vi "Disconnect PV.vi"(8 "Error In":errorcluster, 10 "PV URL":string, 11 "BNT_SLTagMonitor in":refnum<class "BNT_SLTagMonitor.lvclass">) -> (0 "Error Out":errorcluster, 3 "BNT_SLTagMonitor out":refnum<class "BNT_SLTagMonitor.lvclass">)   [LabVIEW 2019, in "BNT_SLTagMonitor.lvlib" / "BNT_SLTagMonitor.lvclass"]
doc: "Close connection to process variable."
uses:
  BNT_SLTagMonitor.lvclass
  CSPP_Core/Actors/CSPP_PVMonitor/CSPP_PVMonitor.lvclass
  <vilib>/Skyline/Tag/Wrapper/Wrapper_class/NI Skyline Tag.lvclass
  <vilib>/Skyline/Tag/Wrapper/Wrapper_class/Close Tag (Single).vi
  C:/Users/Holger/Documents/LVP/CSPP/CSPP-Template/Packages/CSPP_Core/Actors/CSPP_PVMonitor/CSPP_PVMonitor.lvclass
  C:/Users/Holger/Documents/LVP/CSPP/CSPP-Template/Packages/CSPP_Core/Actors/CSPP_BaseActor/CSPP_BaseActor.lvclass
  C:/Program Files (x86)/National Instruments/LabVIEW 2019/vi.lib/ActorFramework/Actor/Actor.lvclass
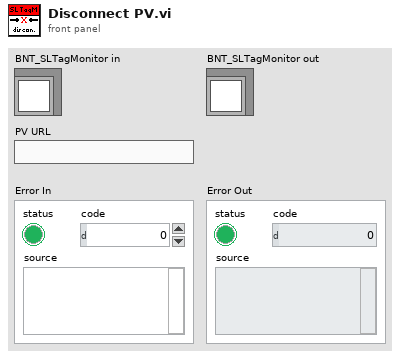
[diagram p1: front panel]
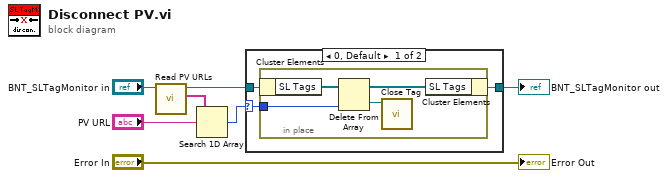
[diagram p0: block diagram]
diagram:
  n1 = call "Read PV URLs.vi"("CSPP_PVMonitor in"="BNT_SLTagMonitor in") -> ("PV URLs"=w6:string[], "CSPP_PVMonitor out"=w3:refnum<class "BNT_SLTagMonitor.lvclass">)  [unwired: 8 in, 1 out]
  n2 = Search 1D Array(1D array=w6, element="PV URL") -> (index of element=w4:i32)  [unwired: 1 in]
  n3 = case shown="0, Default" w4 {
    selector: w4 -> [w10 _]
    tunnel: w3 -> [w9 w15]
    tunnel: [w8 w15] -> w2
    frame 0, Default {
      n4 = in-place {
        in-place-border: w10 -> [w12]
        n5 = in-place-cluster #1(w9) -> ("SL Tags"=w14:refnum<class "NI Skyline Tag.lvclass">[])
        n6 = Delete From Array(array=w14, index=w12) -> (deleted portion=w11:refnum<class "NI Skyline Tag.lvclass">, array with subset deleted=w13:refnum<class "NI Skyline Tag.lvclass">[])  [unwired: 1 in]
        n7 = call-poly <vilib>:"Close Tag.vi"("tag"=w11) -> ()  [unwired: 10 in, 1 out]
        n8 = in-place-cluster #1("SL Tags"=w13) -> (w8:refnum<class "BNT_SLTagMonitor.lvclass">)
      }
    }
    frame -1 {
    }
  }
  "BNT_SLTagMonitor out" <- w2
  "Error Out" <- "Error In"
